vi "Test.vi"   [LabVIEW 2016]
doc: "This VI is called when test mode begins, and will automatically be terminated when it ends. You can add manual or automatic tests and invoke them from the dashboard."
uses:
  Robot Global Data.vi
  <vilib>/Rock Robotics/Network Tables/NT Write Numeric Array.vi
  <vilib>/Rock Robotics/Network Tables/NT Write Raw.vi
  <vilib>/Rock Robotics/Network Tables/NT Write Number.vi
types:
  T1 = typedef "WPI_EncoderDevRef.ctl" = cluster{"DevStatus":errorcluster, "EncoderIndex":T2, "CounterIndex":T3, "DistancePerCount":dbl, "Decoding Type":T4}
  T2 = typedef "FPGA_EncoderIdx.ctl" = enum8{"Enc 0", "Enc 1", "Enc 2", "Enc 3", "Enc 4", "Enc 5", "Enc 6", "Enc 7", "Invalid"}
  T3 = typedef "FPGA_CounterCtrSystemIndex.ctl" = enum8{"Ctr 0", "Ctr 1", "Ctr 2", "Ctr 3", "Ctr 4", "Ctr 5", "Ctr 6", "Ctr 7", "Invalid"}
  T4 = typedef "WPI_EncoderType.ctl" = enum16{"1x", "2x", "4x"}
  T5 = typedef "IMAQ Image.ctl" = refnum<image>
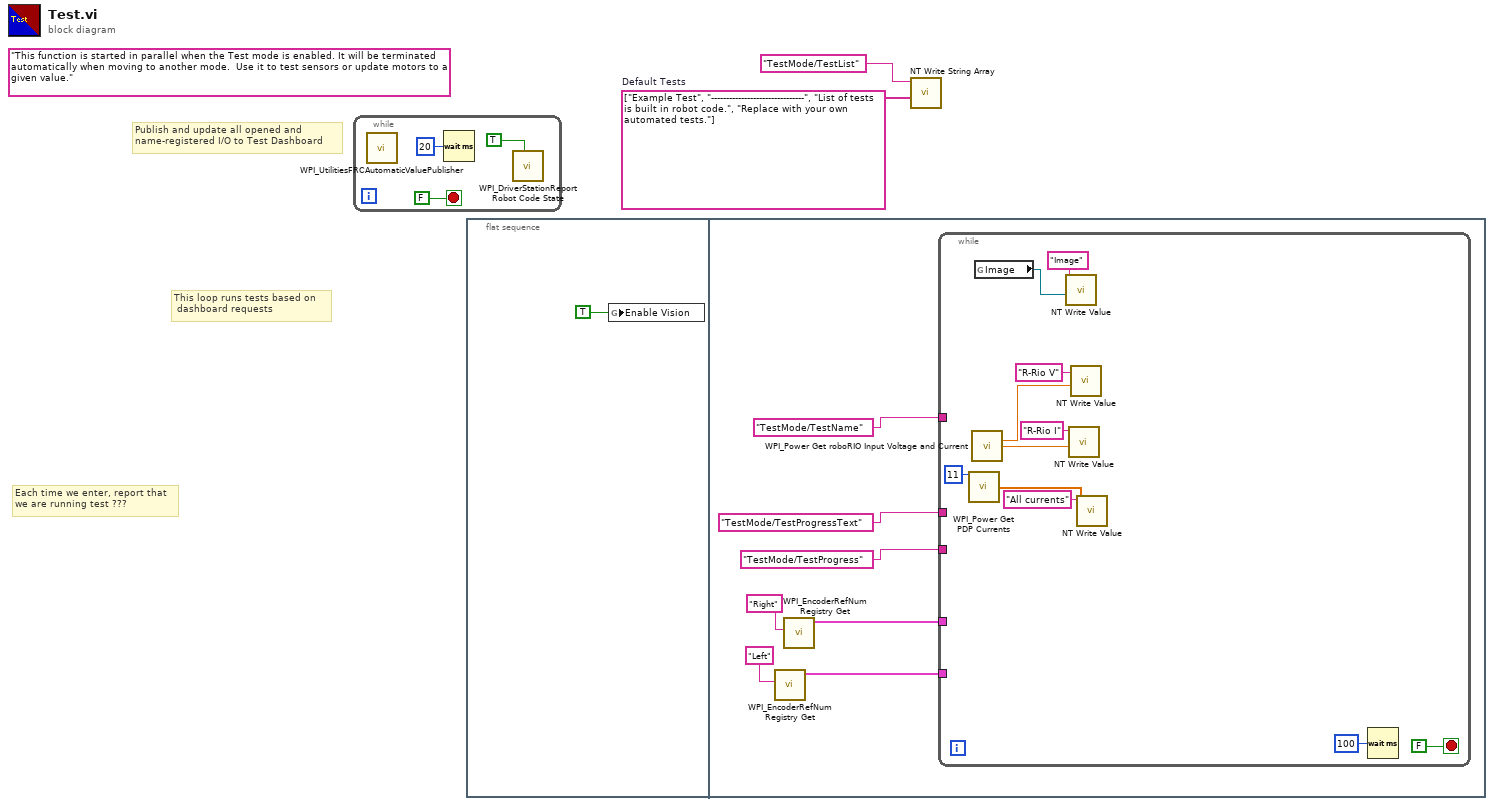
[diagram p0: block diagram]
diagram:
  w2 = string[] ["Example Test", "-------------------------------", "List of tests is built in robot code.", "Replace with your own automated tests."]  # Default Tests
  (unwired) "This function is started in parallel when the Test mode is enabled. It will be terminated automatically when moving to another mode.  Use it to test sensors or update motors to a given value."
  # "This loop runs tests based on \n dashboard requests"
  # "Publish and update all opened and\nname-registered I/O to Test Dashboard"
  # "Each time we enter, report that\nwe are running test ???"
  n1 = while {
    stop <- FALSE stop-if-true
    n2 = call <vilib>:"WPI_UtilitiesFRCAutomaticValuePublisher.vi"() -> ()  [unwired: 12 in]
    n3 = Wait (ms)(milliseconds to wait=u32 20) -> ()  [unwired: 1 out]
    n4 = call <vilib>:"WPI_DriverStationReport Robot Code State.vi"("Test"=TRUE ("Autonomous")) -> ()  [unwired: 10 in, 1 out]
  }
  n5 = flat-sequence {
    frame #0 {
      n6 = global write "Robot Global Data.vi" "Enable Vision"(TRUE) -> ()
    }
    frame #1 {
      n7 = call <vilib>:"WPI_EncoderRefNum Registry Get.vi"("refnum name"="Left") -> ("EncoderDevRef"=w7:T1)  [unwired: 9 in, 1 out]
      n8 = call <vilib>:"WPI_EncoderRefNum Registry Get.vi"("refnum name"="Right") -> ("EncoderDevRef"=w8:T1)  [unwired: 9 in, 1 out]
      n9 = while {
        tunnel: "TestMode/TestName" ("Name") -> [_]
        tunnel: "TestMode/TestProgressText" ("Name") -> [_]
        tunnel: "TestMode/TestProgress" ("Name") -> [_]
        tunnel: w8 -> [_]
        tunnel: w7 -> [_]
        stop <- FALSE stop-if-true
        n10 = call <vilib>:"WPI_Power Get PDP Currents.vi"("Power Distribution Panel (0)"=u8 11) -> ("all currents (A)"=w19:dbl[])  [unwired: 12 in, 2 out]
        n11 = call <vilib>:"WPI_Power Get roboRIO Input Voltage and Current.vi"() -> ("roboRIO input voltage (V)"=w16:dbl, "roboRIO input current (A)"=w17:dbl)  [unwired: 13 in, 1 out]
        n12 = global read "Robot Global Data.vi" "Image"() -> (w22:T5)
        n13 = call-poly <vilib>:"NT Write Value.vi"("Raw"=w22, "Name"="Image") -> ()  [unwired: 9 in, 1 out]
        n14 = call-poly <vilib>:"NT Write Value.vi"("Numeric"=w17, "Name"="R-Rio I") -> ()  [unwired: 9 in, 1 out]
        n15 = call-poly <vilib>:"NT Write Value.vi"("Numeric"=w16, "Name"="R-Rio V") -> ()  [unwired: 9 in, 1 out]
        n16 = call-poly <vilib>:"NT Write Value.vi"("Numeric Array"=w19, "Name"="All currents") -> ()  [unwired: 9 in, 1 out]
        n17 = Wait (ms)(milliseconds to wait=u32 100) -> ()  [unwired: 1 out]
      }
    }
  }
  n18 = call <vilib>:"NT Write String Array.vi"("String Array"=w2, "Name"="TestMode/TestList") -> ()  [unwired: 9 in, 1 out]
